vi "example_GProgramUpload.vi"() -> ()   [LabVIEW 2020]
uses:
  <vilib>/Galil/resources/gclib32/gclib32.lvlib
panel:
  in  "Program":string="#test\nMG TIME\nEN"
  out "Error Out":errorcluster
  in  "IP Address":string="192.168.1.77"
  out "Response":string
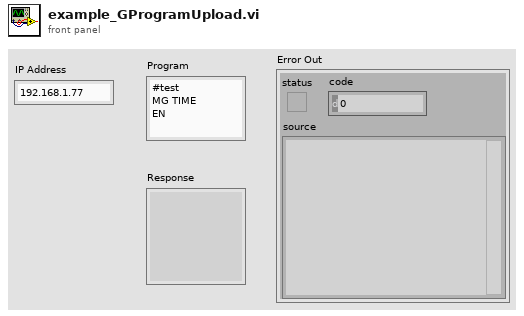
[diagram p1: front panel]
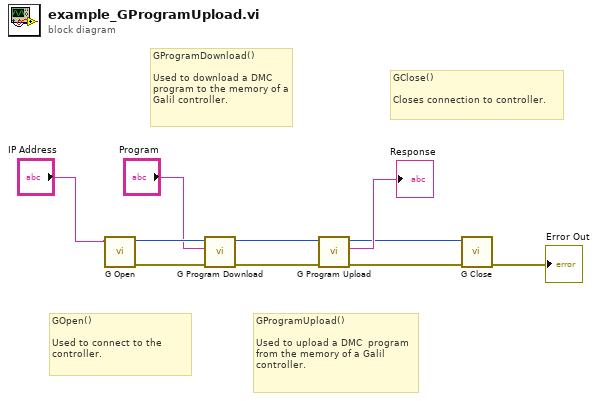
[diagram p0: block diagram]
diagram:
  # "GClose()\n\nCloses connection to controller."
  # "GProgramUpload()\n\nUsed to upload a DMC  program from the memory of a Galil controller."
  # "GProgramDownload()\n\nUsed to download a DMC  program to the memory of a Galil controller."
  # "GOpen()\n\nUsed to connect to the controller."
  n1 = call <vilib>:"G Open.vi"("address"="IP Address") -> ("error out"=w3:errorcluster, "g out"=w5:u32)  [unwired: 8 in]
  n2 = call <vilib>:"G Program Download.vi"("error in (no error)"=w3, "program"="Program", "g"=w5) -> ("error out"=w2:errorcluster, "g out"=w1:u32)  [unwired: 7 in]
  n3 = call <vilib>:"G Program Upload.vi"("error in (no error)"=w2, "g"=w1) -> ("error out"=w6:errorcluster, "buffer out"=→"Response":string, "g out"=w7:u32)  [unwired: 7 in]
  n4 = call <vilib>:"G Close.vi"("error in (no error)"=w6, "g"=w7) -> ("error out"=→"Error Out":errorcluster)  [unwired: 9 in]
